vi "LVClass_HasoEngine ctor from file.vi"(0 "HasoEngine in":refnum<class "HasoEngine.lvclass">, 5 "Configuration file path":path, 11 "error in (no error)":errorcluster) -> (4 "HasoEngine out":refnum<class "HasoEngine.lvclass">, 15 "error out":errorcluster)   [LabVIEW 2020, in "HasoEngine.lvclass"]
doc: "HasoEngine constructor from a Haso configuration file.\n\n--------------------------------------------------------------------------------\n\n<B>HasoEngineIn </B> : Constant Pointer to HasoEngine object.\n<B>HasoEngineOut </B> : Constant Pointer to HasoEngine object.\n<B>config_file_path </B> : Absolute path to Haso configuration file.\n<B>ErrorIn </B> : Error\n<B>ErrorOut </B> : Error\n\n--------------------------------------------------------------------------------"
uses:
  HasoEngine.lvclass
  Handle creation.ctl
  HasoEngine.lvclass/HasoEngine.ctl
  HasoSlopes.lvclass
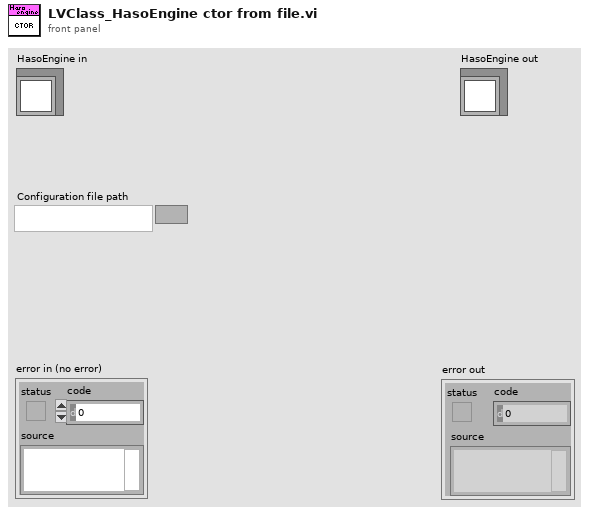
[diagram p1: front panel]
types:
  T1 = typedef "Handle creation.ctl" = enum16{"By ctor", "By write function"}
  T2 = typedef "Point2D.ctl" = cluster{"X":u32, "Y":u32}
  T3 = typedef "Point2Df.ctl" = cluster{"X":sgl, "Y":sgl}
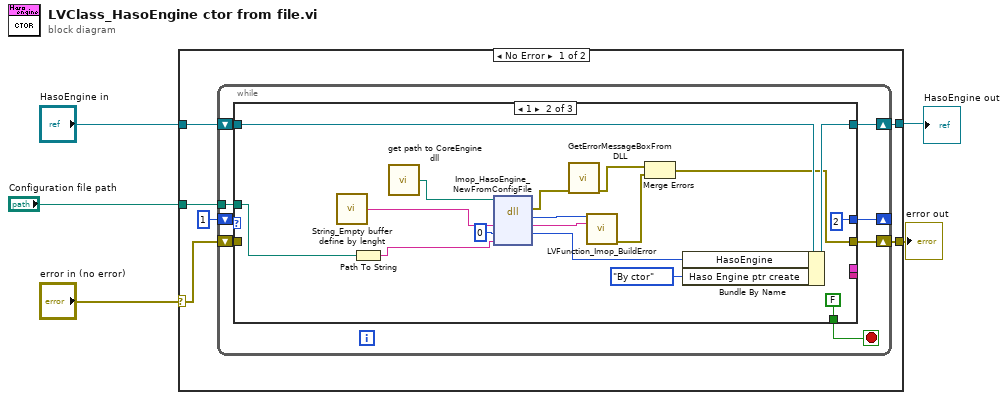
[diagram p0: block diagram]
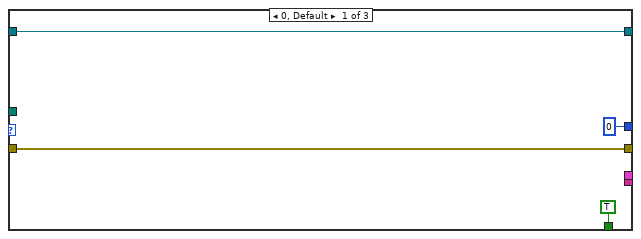
[diagram p2: hidden frame]
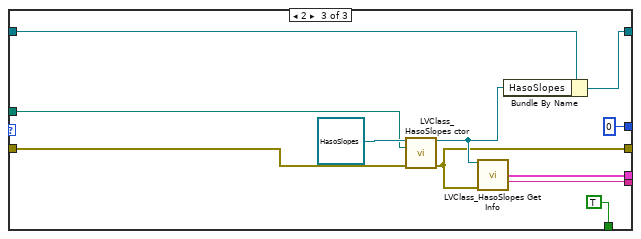
[diagram p3: hidden frame]
diagram:
  n1 = case shown="No Error" "error in (no error)" {
    selector: "error in (no error)" -> [w6 w52]
    tunnel: "HasoEngine in" -> [w11 w53]
    tunnel: [w10 w53] -> w2
    tunnel: [w9 w52] -> w3
    tunnel: "Configuration file path" -> [w7 _]
    frame No Error {
      n2 = while {
        shift-right: [w15] -> _
        shift-left: 1 -> [w16]
        tunnel: w7 -> [w14]
        shift-right: [w17] -> w9
        shift-left: w6 -> [w13]
        shift-right: [w18] -> w10
        shift-left: w11 -> [w19]
        stop <- w12 stop-if-true
        n3 = case shown="1" w16 {
          tunnel: w19 -> [w23 w35 w47]
          tunnel: [w23 w34 w46] -> w18
          tunnel: [w22 w25 w43] -> w17
          tunnel: [0 2 0] -> w15
          tunnel: w14 -> [_ w30 w49]
          tunnel: w13 -> [w22 _ w48]
          tunnel: [TRUE FALSE TRUE] -> w12
          tunnel: [_ _ w42] -> _
          tunnel: [_ _ w41] -> _
          frame 0, Default {
          }
          frame 1 {
            n4 = call "String_Empty buffer define by lenght.vi"() -> ("Empty buffer"=w40:string)  [unwired: 1 in]
            n5 = Path To String(path=w30) -> (string=w29:string)
            n6 = call "get path to CoreEngine dll.vi"() -> ("path to c_interface_vc100.dll"=w24:path)  [unwired: 12 in, 3 out]
            n7 = dll-call lib="D:/soft/HASO_v3/SVN_trunk/ImOpCoreEngine4_LV2011/DLLs/c_interface_vc100.dll" fn="Imop_HasoEngine_NewFromConfigFile"(path in=w24, "message"=w40, "objet"=0, "chemin_config"=w29) -> (error out=w33:errorcluster, "return type"=w37:i32, "message"=w38:string, "objet"=w39:i32)  [unwired: 3 in, 1 out]
            n8 = call "GetErrorMessageBoxFromDLL.vi"("error IN"=w33) -> ("error OUT"=w27:errorcluster)  [unwired: 10 in]
            n9 = call "LVFunction_Imop_BuildError.vi"("code"=w37, "String to Prepend to source (\"\")"=w38) -> ("error out"=w26:errorcluster)  [unwired: 13 in]
            n10 = Merge Errors(w27, w26) -> (w25:errorcluster)
            n11 = Bundle By Name(cluster=w35, "HasoEngine"=w39, "Haso Engine ptr create"=Handle_creation."By ctor") -> (w34:refnum<class "HasoEngine.lvclass">)
          }
          frame 2 {
            n12 = call "LVClass_HasoSlopes ctor.vi"("HasoSlopes in"=refnum<class "HasoSlopes.lvclass"> refnum, "Configuration file path"=w49, "error in (no error)"=w48) -> ("HasoSlopes out"=w44:refnum<class "HasoSlopes.lvclass">, "error out"=w43:errorcluster)  [unwired: 11 in]
            n13 = call "LVClass_HasoSlopes Get Info.vi"("HasoSlopes in"=w44, "error in (no error)"=w43) -> ("dimension"=w41:cluster{"size":T2, "step":T3}, "HASO serial number"=w42:string)  [unwired: 9 in, 3 out]
            n14 = Bundle By Name(cluster=w47, "HasoSlopes"=w44) -> (w46:refnum<class "HasoEngine.lvclass">)
          }
        }
      }
    }
    frame Error {
    }
  }
  "error out" <- w3
  "HasoEngine out" <- w2
